vi "Main.vi"() -> ()   [LabVIEW 2017]
doc: "This Continuous Measurement sample project is based on the Queued Message Handler template.\n\nThe Event Handling Loop generates messages based on user interface actions.\n\nThe Message Handling Loop processes messages generated by the Event Handling Loop, or by other messages. There are also Acquisition and Logging message handling loop subVIs, and a chart updating loop."
uses:
  Settings/Settings.ctl
  Acquisition/Hardware Configuration.ctl
  Acquisition/Signal Type.ctl
  Logging/Logging Configuration.ctl
  controls/UI Data.ctl
  controls/UI State.ctl
  support/Message Queue/Enqueue Message (Single).vi
  controls/ExitGlobal.vi
  support/Message Queue/Enqueue Message (Array).vi
  <vilib>/Utility/error.llb/Error Cluster From Error Code.vi
  <vilib>/ErrorRing/Error Ring.xnode
  Acquisition/Acquisition.lvlib
  Logging/Logging.lvlib
  Settings/Settings.lvlib
  support/User Event - Stop/User Event - Stop.lvlib
  support/Message Queue/Message Queue.lvlib
  Settings/Settings Dialog.vi
panel:
  out "Zero run":bool
  in  "Zero run?":bool
  out "Max writing time to a file [min]":dbl
  out "Test time zero run [s]":dbl
  out "Test time [s]":dbl
  in  "Start":bool
  in  "Stop":bool
  in  "Settings":bool
  out "Status":string
  in  "Exit":bool
  out "Log File Offsite Path":path
  out "Project code":string
  out "Offsite storage?":bool
  out "Log File Path":path
  out "Data":waveform(dbl)[](graph)
  # "Continuous Measurement Data Logger"
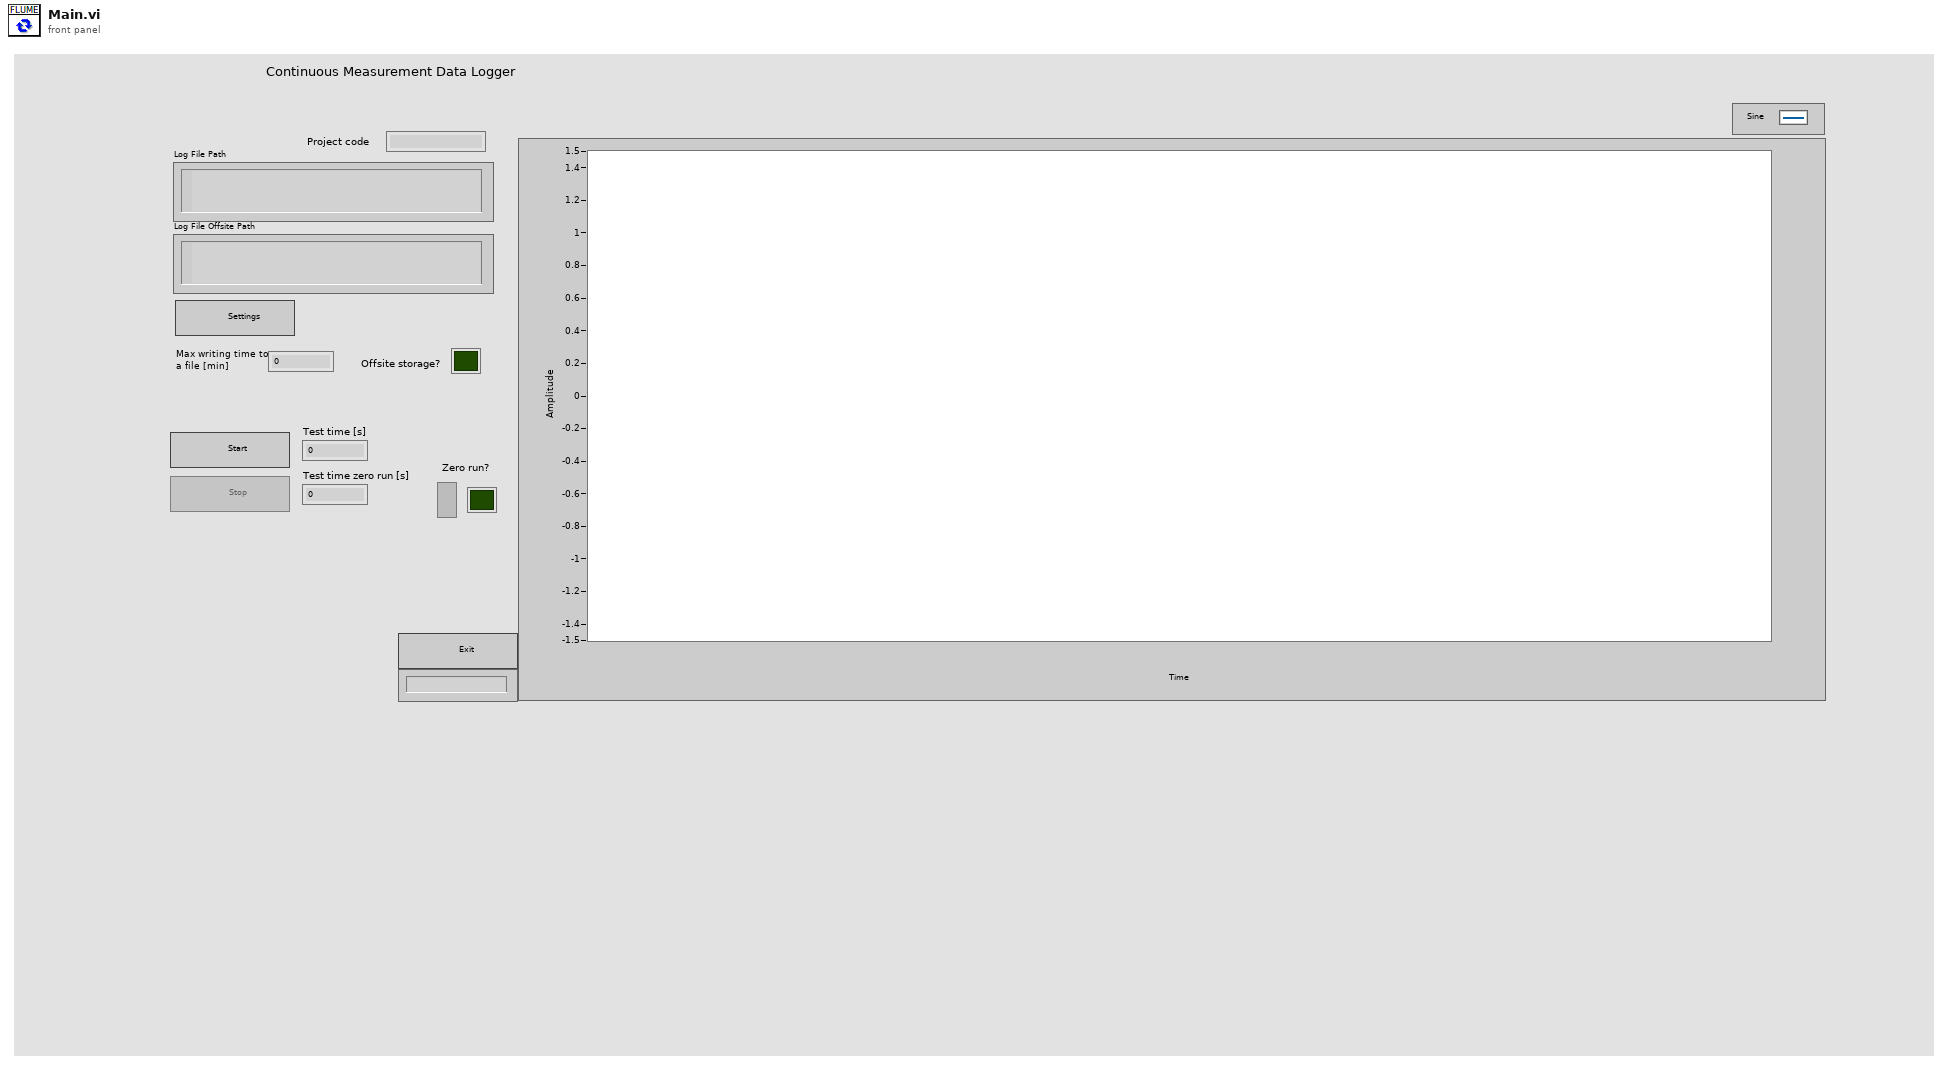
[diagram p1: front panel]
types:
  T1 = cluster{"Offsite storage?":bool, "Test time [s]":dbl, "Test time zero run [s] ":dbl, "Max writing time to a file [min]":dbl, "Zero run":bool}
  T2 = typedef "UI State.ctl" = enum16{"Idle", "Acquiring and Logging", "Waiting for Exit", "Waiting for Exit (Acq Stopped)", "Waiting for Exit (Log Stopped)", "Waiting for Stop", "Waiting for Stop (Acq Stopped)", "Waiting for Stop (Log Stopped)"}
  T3 = typedef "UI Data.ctl" = cluster{"Start Ref":refnum<vi>, "Stop Ref":refnum<vi>, "Settings Ref":refnum<vi>, "Exit Ref":refnum<vi>, "Status Ref":refnum<vi>, "Data Ref":refnum<vi>, "Zero run Ref":refnum<vi>}
  T4 = typedef "Settings.lvlib/Settings.ctl" = cluster{"Hardware Configuration":T5, "Logging Configuration":T7, "Timers":cluster{"Offsite storage?":bool, "Test time [s]":dbl, "Test time zero run [s] ":dbl, "Max writing time to a file [min]":dbl, "Zero run":bool}}
  T5 = typedef "Acquisition.lvlib/Hardware Configuration.ctl" = cluster{"HW Refnum <Replace Me>":string, "Signal Type <Replace Me>":T6}
  T6 = typedef "Acquisition.lvlib/Signal Type.ctl" = enum16{"Sine Wave", "Square with Noise"}
  T7 = typedef "Logging.lvlib/Logging Configuration.ctl" = cluster{"Log File Base Path":path, "TDMS File Reference":refnum<k34>, "Log File Offsite Path":path, "Project code":string, "Bin File Reference":refnum<file>}
  T8 = typedef "Message Queue.lvlib/All Message Queues.ctl" = cluster{"UI":refnum<queue>, "Acquisition":refnum<queue>, "Logging":refnum<queue>, "Bin Logging":refnum<queue>, "Time":refnum<queue>}
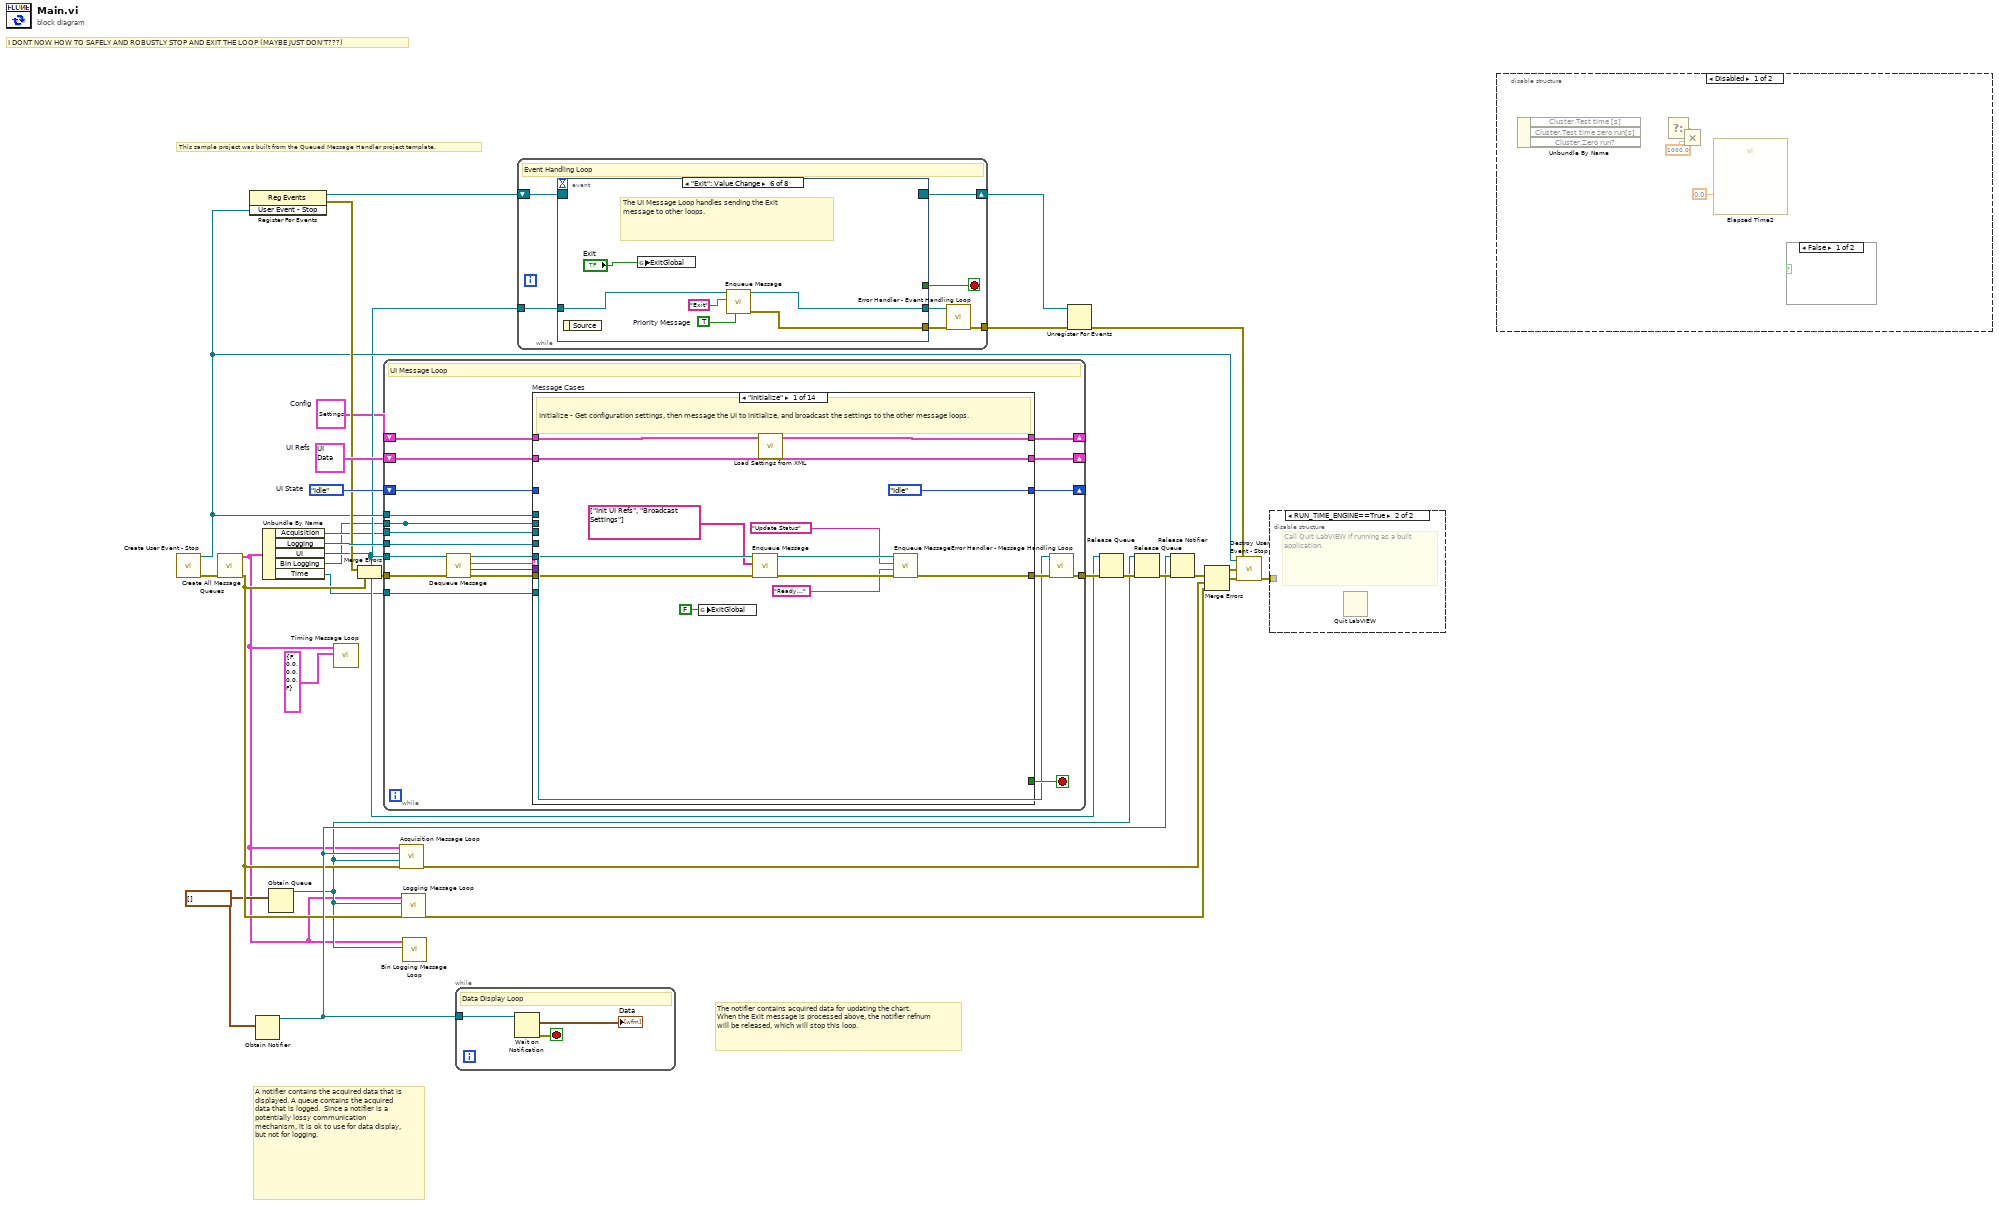
[diagram p0: block diagram]
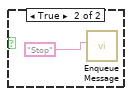
[diagram p2: hidden frame]
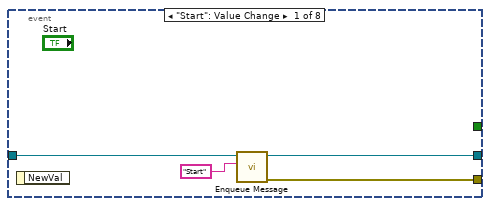
[diagram p5: hidden frame]
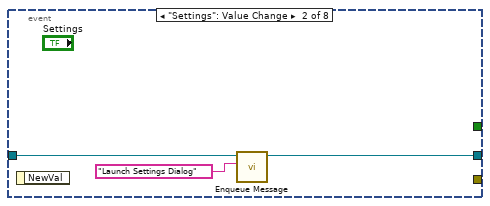
[diagram p6: hidden frame]
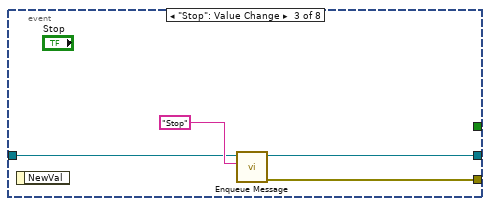
[diagram p7: hidden frame]
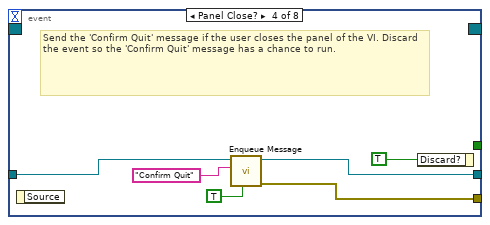
[diagram p8: hidden frame]
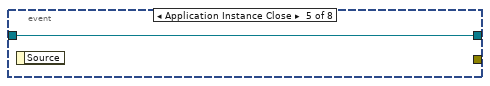
[diagram p9: hidden frame]
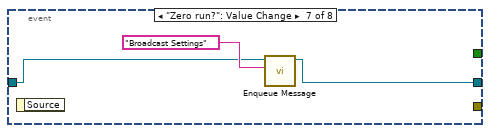
[diagram p10: hidden frame]
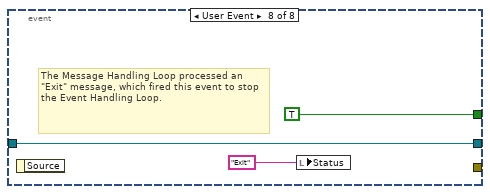
[diagram p11: hidden frame]
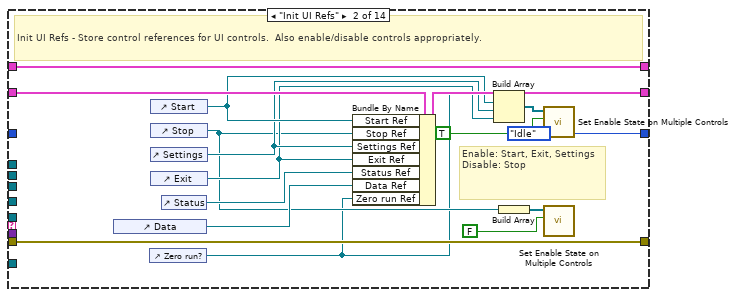
[diagram p12: hidden frame]
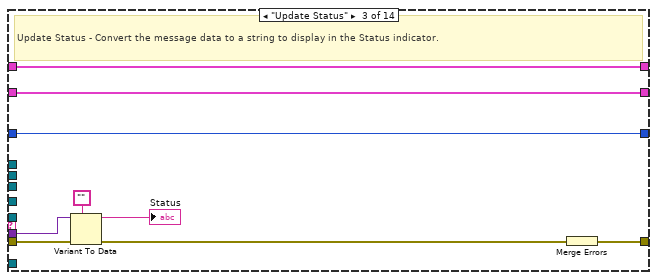
[diagram p13: hidden frame]
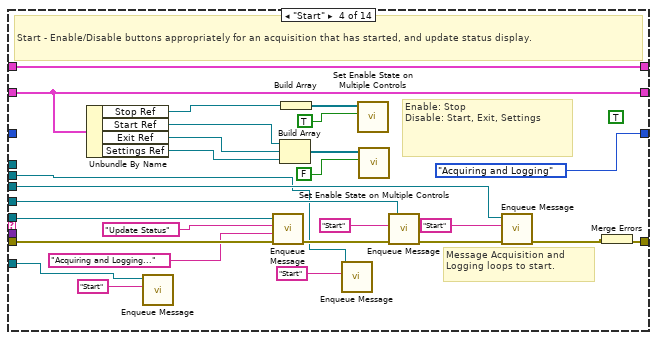
[diagram p14: hidden frame]
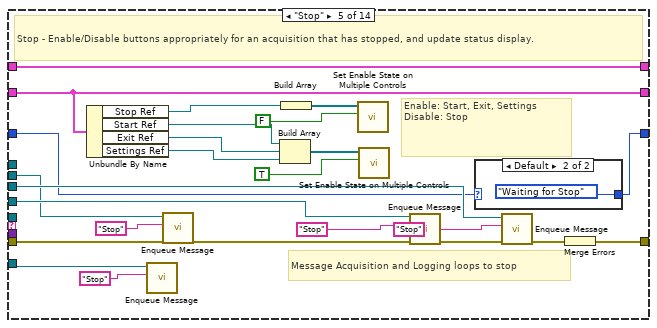
[diagram p15: hidden frame]
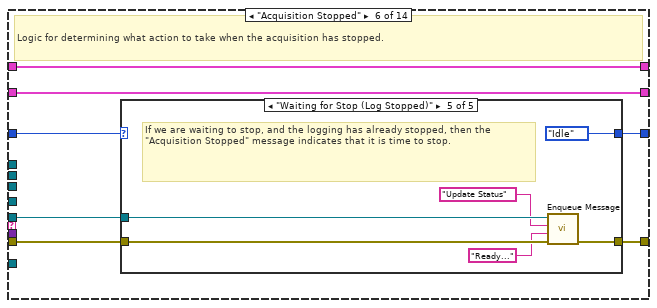
[diagram p17: hidden frame]
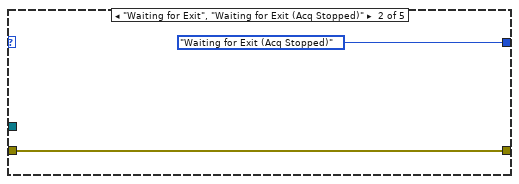
[diagram p19: hidden frame]
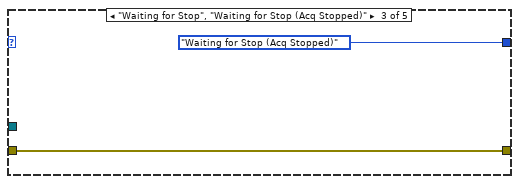
[diagram p20: hidden frame]
diagram:
  w23 = UI_State."Idle"  # UI State
  w7 = waveform(dbl)[] []
  w25 = T3 {"Start Ref"=refnum, "Stop Ref"=refnum, "Settings Ref"=refnum, "Exit Ref"=refnum, "Status Ref"=refnum, "Data Ref"=refnum, "Zero run Ref"=refnum}  # UI Refs
  w9 = T4 {"Hardware Configuration"={"HW Refnum <Replace Me>"="", "Signal Type <Replace Me>"=enum."Sine Wave"}, "Logging Configuration"={"Log File Base Path"=path "", "TDMS File Reference"=refnum, "Log File Offsite Path"=path "", "Project code"="", "Bin File Reference"=refnum}, "Timers"={"Offsite storage?"=FALSE, "Test time [s]"=10.0, "Test time zero run [s] "=180.0, "Max writing time to a file [min]"=30.0, "Zero run"=FALSE}}  # Config
  # "I DONT NOW HOW TO SAFELY AND ROBUSTLY STOP AND EXIT THE LOOP (MAYBE JUST DON'T???)"
  # "This sample project was built from the Queued Message Handler project template."
  # "A notifier contains the acquired data that is displayed. A queue contains the acquired data that is logged.  Since a notifier is a potentially lossy communication mechanism, it is ok to use for data display, but not for logging."
  # "The notifier contains acquired data for updating the chart. When the Exit message is processed above, the notifier refnum will be released, which will stop this loop."
  n1 = call "Create User Event - Stop.vi"() -> ("error out"=w27:errorcluster, "User Event - Stop"=w14:refnum<user-event>)  [unwired: 10 in]
  n2 = call "Create All Message Queues.vi"("error in (no error)"=w27) -> ("error out"=w8:errorcluster, "Message Queues out"=w2:T8)  [unwired: 9 in]
  n3 = register-events(w14) -> (reference out=w17:refnum<event-registration>, error out=w15:errorcluster)  [unwired: 2 in]
  n4 = Obtain Notifier(notification data type=w7) -> (notifier out=w10:refnum<notifier>)  [unwired: 3 in, 2 out]
  n5 = Unbundle By Name(w2) -> ("Acquisition"=w12:refnum<queue>, "Logging"=w24:refnum<queue>, "UI"=w13:refnum<queue>, "Bin Logging"=w5:refnum<queue>, "Time"=w1:refnum<queue>)
  n6 = Obtain Queue(element data type=w7) -> (queue out=w6:refnum<queue>)  [unwired: 4 in, 2 out]
  n7 = call "Timing Message Loop.vi"("Timers"=T1 {"Offsite storage?"=FALSE, "Test time [s]"=0.0, "Test time zero run [s] "=0.0, "Max writing time to a file [min]"=0.0, "Zero run"=FALSE}, "Message Queues"=w2) -> ()  [unwired: 9 in, 1 out]
  n8 = Merge Errors(w15, w8) -> (w16:errorcluster)
  n9 = while {
    tunnel: w13 -> [w36]
    tunnel: w14 -> [w49]
    shift-right: [w44] -> _
    shift-left: w9 -> [w32]
    shift-right: [w42] -> _
    shift-left: w25 -> [w43]
    tunnel: w12 -> [w41]
    tunnel: w24 -> [w35]
    shift-right: [w37] -> _
    shift-left: w23 -> [w38]
    tunnel: w16 -> [w48]
    tunnel: [w40] -> w30
    tunnel: w5 -> [w33]
    tunnel: [w33] -> _
    tunnel: w1 -> [w31]
    stop <- w50 stop-if-true
    # "UI Message Loop"
    n10 = call "Dequeue Message.vi"("error in (no error)"=w48, "Message Queue"=w36) -> ("error out"=w47:errorcluster, "Message Data"=w45:variant, "Message"=w46:string, "dup Message Queue"=w34:refnum<queue>)  [unwired: 6 in]
    n11 = case "Message Cases" shown="\"Initialize\"" w46 {
      selector: w46 -> [_ _ _ _ _ _ _ _ _ _ _ _ _ w295]
      tunnel: w34 -> [w56 _ _ w94 _ w145 w170 _ w223 _ w245 _ _ _]
      tunnel: w47 -> [w55 w79 w87 w115 w138 w146 w171 w213 w225 w233 w244 w279 w293 _]
      tunnel: [w60 w79 w88 w96 w139 w143 w168 w217 w219 w236 w243 w286 w292 w294] -> w39
      tunnel: [_ _ _ _ _ _ _ _ _ _ _ TRUE _ _] -> w50
      tunnel: w45 -> [_ _ w86 _ _ _ _ _ _ w237 _ w277 _ _]
      tunnel: w49 -> [_ _ _ _ _ _ _ _ _ _ _ w287 _ _]
      tunnel: [w63 w66 w80 w92 w120 w142 w167 w196 w218 w232 w241 w275 w291 w298] -> w44
      tunnel: w32 -> [w52 w66 w80 w92 w120 w142 w167 w201 w226 w232 w241 w275 w291 w298]
      tunnel: w43 -> [w57 w78 w82 w112 w137 w148 w173 w212 w221 w240 w247 w285 w290 w297]
      tunnel: [w57 w75 w82 w112 w137 w148 w173 w212 w221 w240 w247 w285 w290 w297] -> w42
      tunnel: w41 -> [_ _ _ w95 w124 _ _ w211 _ _ _ w284 _ _]
      tunnel: w35 -> [_ _ _ w101 w127 _ _ w210 _ _ _ w283 _ _]
      tunnel: w38 -> [_ _ w81 _ w121 w147 w172 w209 w220 w235 w246 _ w289 w296]
      tunnel: [UI_State."Idle" ("UI State") UI_State."Idle" ("UI State") w81 UI_State."Acquiring and Logging" ("UI State") w122 w144 w169 w209 w220 w235 w242 UI_State."Idle" ("UI State") w289 w296] -> w37
      tunnel: w33 -> [_ _ _ w91 w118 _ _ w204 _ _ _ w274 _ _]
      tunnel: w31 -> [_ _ _ w89 w117 _ _ w200 _ _ _ w270 _ _]
      frame "Initialize" {
        # "Initialize - Get configuration settings, then message the UI to initialize, and broadcast the settings to the other message loops."
        n12 = global write "ExitGlobal.vi" "ExitGlobal"(FALSE ("ExitGlobal")) -> ()
        n13 = call-poly "Enqueue Message.vi"("error in (no error)"=w55, "Message Array"=string[] ["Init UI Refs", "Broadcast Settings"], "Message Queue"=w56) -> ("error out"=w62:errorcluster, "dup Message Queue"=w61:refnum<queue>)  [unwired: 7 in]
        n14 = call "Load Settings from XML.vi"("Settings in"=w52) -> ("Settings out"=w63:T4)  [unwired: 9 in, 1 out]
        n15 = call-poly "Enqueue Message.vi"("error in (no error)"=w62, "Message Data"="Ready..." ("Ready..."), "Message"="Update Status", "Message Queue"=w61) -> ("error out"=w60:errorcluster)  [unwired: 6 in, 1 out]
      }
      frame "Init UI Refs" {
        # "Enable: Start, Exit, Settings\nDisable: Stop"
        # "Init UI Refs - Store control references for UI controls.  Also enable/disable controls appropriately."
        n16 = control-ref of="Data"() -> (w76:refnum<vi>)
        n17 = control-ref of="Zero run?"() -> (w64:refnum<vi>)
        n18 = control-ref of="Start"() -> (w70:refnum<vi>)
        n19 = control-ref of="Stop"() -> (w65:refnum<vi>)
        n20 = control-ref of="Settings"() -> (w69:refnum<vi>)
        n21 = control-ref of="Exit"() -> (w68:refnum<vi>)
        n22 = control-ref of="Status"() -> (w77:refnum<vi>)
        n23 = Bundle By Name(cluster=w78, "Start Ref"=w70, "Stop Ref"=w65, "Settings Ref"=w69, "Exit Ref"=w68, "Status Ref"=w77, "Data Ref"=w76, "Zero run Ref"=w64) -> (w75:T3)
        n24 = Build Array(w64, w70, w69, w68) -> (w73:refnum<vi>[])
        n25 = Build Array(w65) -> (w72:refnum<vi>[])
        n26 = call "Set Enable State on Multiple Controls.vi"("Enable?"=TRUE, "Controls"=w73) -> ()  [unwired: 10 in]
        n27 = call "Set Enable State on Multiple Controls.vi"("Enable?"=FALSE, "Controls"=w72) -> ()  [unwired: 10 in]
      }
      frame "Update Status" {
        # "Update Status - Convert the message data to a string to display in the Status indicator."
        n28 = Variant To Data(error in=w87, type="", Variant=w86) -> (data=→"Status":string, error out=w84:errorcluster)
        n29 = Merge Errors(w84) -> (w88:errorcluster)
      }
      frame "Start" {
        (unwired) TRUE ("Reset")
        # "Message Acquisition and Logging loops to start."
        # "Enable: Stop\nDisable: Start, Exit, Settings"
        # "Start - Enable/Disable buttons appropriately for an acquisition that has started, and update status display."
        n30 = Unbundle By Name(w112) -> ("Stop Ref"=w107:refnum<vi>, "Start Ref"=w106:refnum<vi>, "Exit Ref"=w105:refnum<vi>, "Settings Ref"=w104:refnum<vi>)
        n31 = call-poly "Enqueue Message.vi"("Message"="Start", "Message Queue"=w89) -> ()  [unwired: 8 in, 2 out]
        n32 = call-poly "Enqueue Message.vi"("error in (no error)"=w115, "Message Data"="Acquiring and Logging..." ("Acquiring and Logging..."), "Message"="Update Status", "Message Queue"=w94) -> ("error out"=w103:errorcluster)  [unwired: 6 in, 1 out]
        n33 = Build Array(w106, w105, w104) -> (w110:refnum<vi>[])
        n34 = Build Array(w107) -> (w109:refnum<vi>[])
        n35 = call-poly "Enqueue Message.vi"("Message"="Start", "Message Queue"=w91) -> ()  [unwired: 8 in, 2 out]
        n36 = call "Set Enable State on Multiple Controls.vi"("Enable?"=TRUE, "Controls"=w109) -> ()  [unwired: 10 in]
        n37 = call "Set Enable State on Multiple Controls.vi"("Enable?"=FALSE, "Controls"=w110) -> ()  [unwired: 10 in]
        n38 = call-poly "Enqueue Message.vi"("error in (no error)"=w103, "Message"="Start", "Message Queue"=w101) -> ("error out"=w98:errorcluster)  [unwired: 7 in, 1 out]
        n39 = call-poly "Enqueue Message.vi"("error in (no error)"=w98, "Message"="Start", "Message Queue"=w95) -> ("error out"=w97:errorcluster)  [unwired: 7 in, 1 out]
        n40 = Merge Errors(w97) -> (w96:errorcluster)
      }
      frame "Stop" {
        # "Message Acquisition and Logging loops to stop"
        # "Enable: Start, Exit, Settings\nDisable: Stop"
        # "Stop - Enable/Disable buttons appropriately for an acquisition that has stopped, and update status display."
        n41 = Unbundle By Name(w137) -> ("Stop Ref"=w132:refnum<vi>, "Start Ref"=w131:refnum<vi>, "Exit Ref"=w130:refnum<vi>, "Settings Ref"=w129:refnum<vi>)
        n42 = call-poly "Enqueue Message.vi"("Message"="Stop", "Message Queue"=w117) -> ()  [unwired: 8 in, 2 out]
        n43 = call-poly "Enqueue Message.vi"("Message"="Stop", "Message Queue"=w118) -> ()  [unwired: 8 in, 2 out]
        n44 = Build Array(w131, w130, w129) -> (w135:refnum<vi>[])
        n45 = Build Array(w132) -> (w134:refnum<vi>[])
        n46 = call "Set Enable State on Multiple Controls.vi"("Enable?"=FALSE, "Controls"=w134) -> ()  [unwired: 10 in]
        n47 = call "Set Enable State on Multiple Controls.vi"("Enable?"=TRUE, "Controls"=w135) -> ()  [unwired: 10 in]
        n48 = call-poly "Enqueue Message.vi"("error in (no error)"=w138, "Message"="Stop", "Message Queue"=w127) -> ("error out"=w126:errorcluster)  [unwired: 7 in, 1 out]
        n49 = case shown="Default" w121 {
          selector: w121 -> [w140 _]
          tunnel: [w140 UI_State."Waiting for Stop" ("UI State")] -> w122
          frame "Waiting for Exit" {
          }
          frame Default {
          }
        }
        n50 = call-poly "Enqueue Message.vi"("error in (no error)"=w126, "Message"="Stop", "Message Queue"=w124) -> ("error out"=w125:errorcluster)  [unwired: 7 in, 1 out]
        n51 = Merge Errors(w125) -> (w139:errorcluster)
      }
      frame "Acquisition Stopped" {
        # "Logic for determining what action to take when the acquisition has stopped."
        n52 = case shown="\"Waiting for Stop (Log Stopped)\"" w147 {
          selector: w147 -> [w150 _ _ _ _]
          tunnel: w146 -> [w149 w152 w154 w160 w166]
          tunnel: w145 -> [_ _ _ w158 w163]
          tunnel: [w150 UI_State."Waiting for Exit (Acq Stopped)" ("UI State") UI_State."Waiting for Stop (Acq Stopped)" ("UI State") UI_State."Idle" ("UI State") UI_State."Idle" ("UI State")] -> w144
          tunnel: [w149 w152 w154 w159 w164] -> w143
          frame Default {
          }
          frame "Waiting for Exit", "Waiting for Exit (Acq Stopped)" {
          }
          frame "Waiting for Stop", "Waiting for Stop (Acq Stopped)" {
          }
          frame "Waiting for Exit (Log Stopped)" {
            # "If we are waiting to exit, and the logging has already stopped, then the \"Acquisition Stopped\" message indicates that it is time to exit."
            n53 = call-poly "Enqueue Message.vi"("Priority Message? (F)"=TRUE, "error in (no error)"=w160, "Message"="Exit", "Message Queue"=w158) -> ("error out"=w159:errorcluster)  [unwired: 6 in, 1 out]
          }
          frame "Waiting for Stop (Log Stopped)" {
            # "If we are waiting to stop, and the logging has already stopped, then the \"Acquisition Stopped\" message indicates that it is time to stop."
            n54 = call-poly "Enqueue Message.vi"("error in (no error)"=w166, "Message Data"="Ready..." ("Ready..."), "Message"="Update Status", "Message Queue"=w163) -> ("error out"=w164:errorcluster)  [unwired: 6 in, 1 out]
          }
        }
      }
      frame "Logging Stopped" {
        # "Logic for determining what action to take when the logging has stopped."
        n55 = case shown="Default" w172 {
          selector: w172 -> [w175 _ _ _ _]
          tunnel: w171 -> [w174 w177 w179 w185 w188]
          tunnel: w170 -> [_ _ _ w183 w187]
          tunnel: [w175 UI_State."Waiting for Exit (Log Stopped)" ("UI State") UI_State."Waiting for Stop (Log Stopped)" ("UI State") UI_State."Idle" ("UI State") UI_State."Idle" ("UI State")] -> w169
          tunnel: [w174 w177 w179 w184 w186] -> w168
          frame Default {
          }
          frame "Waiting for Exit", "Waiting for Exit (Log Stopped)" {
          }
          frame "Waiting for Stop", "Waiting for Stop (Log Stopped)" {
          }
          frame "Waiting for Exit (Acq Stopped)" {
            # "If we are waiting to exit, and the acquisition has already stopped, then the \"Logging Stopped\" message indicates that it is time to exit."
            n56 = call-poly "Enqueue Message.vi"("Priority Message? (F)"=TRUE, "error in (no error)"=w185, "Message"="Exit", "Message Queue"=w183) -> ("error out"=w184:errorcluster)  [unwired: 6 in, 1 out]
          }
          frame "Waiting for Stop (Acq Stopped)" {
            # "If we are waiting to stop, and the acquisition has already stopped, then the \"Logging Stopped\" message indicates that it is time to stop."
            n57 = call-poly "Enqueue Message.vi"("error in (no error)"=w188, "Message Data"="Ready..." ("Ready..."), "Message"="Update Status", "Message Queue"=w187) -> ("error out"=w186:errorcluster)  [unwired: 6 in, 1 out]
          }
        }
      }
      frame "Broadcast settings" {
        w199 = "Update Settings" ("Message")
        # "Broadcast settings - Send the 'Update Settings' message to the Logging and Acquisition message loops."
        n58 = Unbundle By Name(w201) -> ("Hardware Configuration"=w215:T5, "Logging Configuration"=w203:T7, "Timers"=w198:T1)
        n59 = Unbundle By Name(w203) -> ("Log File Base Path"=→"Log File Path":path, "Log File Offsite Path"=→"Log File Offsite Path":path, "Project code"=→"Project code":string)
        n60 = Bundle By Name(cluster=w201, "Timers.Zero run"="Zero run?") -> (w196:T4)
        n61 = Unbundle By Name(w198) -> ("Max writing time to a file [min]"=→"Max writing time to a file [min]":dbl, "Offsite storage?"=→"Offsite storage?":bool, "Test time [s]"=→"Test time [s]":dbl, "Test time zero run [s]"=→"Test time zero run [s]":dbl)
        n62 = Unbundle By Name(w196) -> ("Timers"=w195:T1)
        n63 = call-poly "Enqueue Message.vi"("Message Data"=w215, "Message"=w199, "Message Queue"=w211) -> ("error out"=w216:errorcluster)  [unwired: 7 in, 1 out]
        n64 = call-poly "Enqueue Message.vi"("Message Data"=w195, "Message"=w199, "Message Queue"=w200) -> ("error out"=w194:errorcluster)  [unwired: 7 in, 1 out]
        n65 = call-poly "Enqueue Message.vi"("Message Data"=w203, "Message"=w199, "Message Queue"=w204) -> ()  [unwired: 7 in, 2 out]
        n66 = call-poly "Enqueue Message.vi"("error in (no error)"=w216, "Message Data"=w203, "Message"=w199, "Message Queue"=w210) -> ("error out"=w214:errorcluster)  [unwired: 6 in, 1 out]
        n67 = Merge Errors(w214, w213, w194) -> (w217:errorcluster)
        "Zero run" <- "Zero run?"
      }
      frame "Launch Settings Dialog" {
        # "Launch Settings Dialog - Launch the Settings Dialog when the user clicks the 'Settings' button."
        n68 = call-by-ref "?"("error in (no error)"=w225, "Settings in"=w226) -> ("error out"=w222:errorcluster, "Cancelled?"=w224:bool, "Settings out"=w218:T4)  [unwired: 8 in, 3 out]
        n69 = case shown="False" w224 {
          tunnel: w223 -> [w230 _]
          tunnel: w222 -> [w229 w231]
          tunnel: [w228 w231] -> w219
          frame False {
            n70 = call-poly "Enqueue Message.vi"("error in (no error)"=w229, "Message"="Broadcast Settings", "Message Queue"=w230) -> ("error out"=w228:errorcluster)  [unwired: 7 in, 1 out]
          }
          frame True {
          }
        }
      }
      frame "Error" {
        # "Error - Display an error dialog. This message is sent by the \"Error Handler\" VIs at the end of other loops in this application."
        n71 = Variant To Data(error in=w233, type=errorcluster {"status"=FALSE, "code"=0, "source"=""} ("error constant"), Variant=w237) -> (data=w234:errorcluster, error out=w238:errorcluster)
        n72 = call <vilib>:"Simple Error Handler.vi"("error in (no error)"=w234) -> ()  [unwired: 4 in, 5 out]
        n73 = Merge Errors(w238) -> (w236:errorcluster)
      }
      frame "Confirm Quit" {
        # "Confirm Quit - Message that can confirm whether or not the user wants to exit the application."
        n74 = case shown="\"Acquiring and Logging\"" w246 {
          tunnel: w245 -> [w253 w257]
          tunnel: w244 -> [w252 w256]
          tunnel: [w251 w255] -> w243
          tunnel: [UI_State."Idle" ("UI State") w254] -> w242
          frame Default {
            # "If 'Confirm Quit' comes in while the system is idle, there is no need for a confirmation message."
            n75 = call-poly "Enqueue Message.vi"("Priority Message? (F)"=TRUE, "error in (no error)"=w252, "Message"="Exit", "Message Queue"=w253) -> ("error out"=w251:errorcluster)  [unwired: 6 in, 1 out]
          }
          frame "Acquiring and Logging" {
            n76 = Two Button Dialog(message="Are you sure you want to quit while the acquisition is running?" ("Confirm Quit Message"), 1:"No" ("No"), 2:"Yes" ("Yes")) -> (T button?=w258:bool)
            n77 = case shown="True" w258 {
              tunnel: w257 -> [_ w267]
              tunnel: w256 -> [w263 w268]
              tunnel: [w263 w266] -> w255
              tunnel: [UI_State."Acquiring and Logging" ("UI State") UI_State."Waiting for Exit" ("UI State")] -> w254
              frame False {
                # "User did not want to quit."
              }
              frame True {
                n78 = call-poly "Enqueue Message.vi"("error in (no error)"=w268, "Message"="Stop", "Message Queue"=w267) -> ("error out"=w266:errorcluster)  [unwired: 7 in, 1 out]
              }
            }
          }
        }
      }
      frame "Exit" {
        w280 = TRUE ("Priority Message? (F)")
        w273 = "Exit" ("Message")
        # "Popup an error dialog if 'Exit' was called as a result of an error."
        # "Stop the VI"
        # "Exit - Send Exit messages to the Acquisition and Logging loops, and fire the user event to stop the Event Handling Loop."
        n79 = call-poly "Enqueue Message.vi"("Message"="Exit", "Message Queue"=w270) -> ()  [unwired: 8 in, 2 out]
        n80 = Variant To Data(type=errorcluster {"status"=FALSE, "code"=0, "source"=""} ("error constant"), Variant=w277) -> (data=w276:errorcluster)  [unwired: 1 in, 1 out]
        n81 = call <vilib>:"Simple Error Handler.vi"("error in (no error)"=w276) -> ()  [unwired: 4 in, 5 out]
        n82 = call-poly "Enqueue Message.vi"("Priority Message? (F)"=w280, "error in (no error)"=w279, "Message"=w273, "Message Queue"=w284) -> ("error out"=w281:errorcluster)  [unwired: 6 in, 1 out]
        n83 = call-poly "Enqueue Message.vi"("Priority Message? (F)"=w280, "error in (no error)"=w281, "Message"=w273, "Message Queue"=w283) -> ("error out"=w272:errorcluster)  [unwired: 6 in, 1 out]
        n84 = call-poly "Enqueue Message.vi"("error in (no error)"=w272, "Message"=w273, "Message Queue"=w274) -> ("error out"=w271:errorcluster)  [unwired: 7 in, 1 out]
        n85 = call "Fire User Event - Stop.vi"("error in (no error)"=w271, "User Event - Stop"=w287) -> ("error out"=w286:errorcluster)  [unwired: 9 in]
      }
      frame "---Copy This Frame---" {
        (unwired) FALSE ("Time has Elapsed")
        # "Duplicate this frame when creating new messages.  Change this comment in the duplicated frame to describe this message."
        n86 = Merge Errors(w293) -> (w292:errorcluster)
      }
      frame Default {
        # "'Default' case only runs if there is a message that isn't defined in any of the other cases.  Output a programming error."
        n87 = xnode "Error Ring"("parameter 0"=w295) -> ("error out"=w294:errorcluster)
      }
    }
    n88 = call "Error Handler - Message Handling Loop.vi"("error in (no error)"=w39, "Message Queue"=w34) -> ("dup error in"=w40:errorcluster)  [unwired: 8 in, 1 out]
  }
  n89 = call "Acquisition Message Loop.vi"("error in (no error)"=w8, "Data Queue"=w6, "Data Notifier"=w10, "Message Queues"=w2) -> ("error out"=w28:errorcluster)  [unwired: 7 in]
  n90 = call "Logging Message Loop.vi"("error in (no error)"=w8, "Data Queue"=w6, "Message Queues"=w2) -> ("error out"=w4:errorcluster)  [unwired: 8 in]
  n91 = call "Bin Logging Message Loop.vi"("Data Queue"=w6, "Message Queues"=w2) -> ()  [unwired: 9 in, 1 out]
  n92 = while "Data Display Loop" {
    tunnel: w10 -> [w308]
    stop <- w307 stop-if-true
    # "Data Display Loop"
    n93 = Wait on Notification(notifier=w308) -> (notification=→"Data":waveform(dbl)[], error out=w307:errorcluster)  [unwired: 3 in, 2 out]
  }
  n94 = while {
    tunnel: w13 -> [w314]
    tunnel: [w311] -> w29
    shift-right: [w313] -> w26
    shift-left: w17 -> [w315]
    stop <- w312 stop-if-true
    # "Event Handling Loop"
    n95 = event shown="[5] \"Exit\": Value Change" {
      selector: w315 -> [_ _ _ _ _ _ _ _]
      dyn-events: [_ _ _ _ _ _ _ _] -> w313
      timeout: _ -> [_ _ _ _ _ _ _ _]
      tunnel: [_ _ _ _ _ _ _ TRUE ("Discard?")] -> w312
      tunnel: w314 -> [w319 w321 w325 w330 w333 w336 w341 w343]
      tunnel: [w317 _ w324 w328 _ w339 _ _] -> w310
      tunnel: [w316 w320 w323 w329 w333 w335 w340 w343] -> w309
      event "Start": Value Change {
        n96 = event-data() -> ()  [unwired: 1 in, 1 out]
        n97 = call-poly "Enqueue Message.vi"("Message"="Start", "Message Queue"=w319) -> ("error out"=w317:errorcluster, "dup Message Queue"=w316:refnum<queue>)  [unwired: 8 in]
      }
      event "Settings": Value Change {
        n98 = event-data() -> ()  [unwired: 1 in, 1 out]
        n99 = call-poly "Enqueue Message.vi"("Message"="Launch Settings Dialog", "Message Queue"=w321) -> ("dup Message Queue"=w320:refnum<queue>)  [unwired: 8 in, 1 out]
      }
      event "Stop": Value Change {
        n100 = event-data() -> ()  [unwired: 1 in, 1 out]
        n101 = call-poly "Enqueue Message.vi"("Message"="Stop", "Message Queue"=w325) -> ("error out"=w324:errorcluster, "dup Message Queue"=w323:refnum<queue>)  [unwired: 8 in]
      }
      event Panel Close? {
        # "Send the 'Confirm Quit' message if the user closes the panel of the VI. Discard the event so the 'Confirm Quit' message has a chance to run."
        n102 = event-data() -> ()  [unwired: 1 in, 1 out]
        n103 = call-poly "Enqueue Message.vi"("Priority Message? (F)"=TRUE, "Message"="Confirm Quit", "Message Queue"=w330) -> ("error out"=w328:errorcluster, "dup Message Queue"=w329:refnum<queue>)  [unwired: 7 in]
        n104 = event-data("Discard?"=TRUE) -> ()  [unwired: 1 in, 1 out]
      }
      event Application Instance Close {
        n105 = event-data() -> ()  [unwired: 1 in, 1 out]
      }
      event "Exit": Value Change {
        w337 = TRUE  # Priority Message
        # "The UI Message Loop handles sending the Exit message to other loops."
        n106 = event-data() -> ()  [unwired: 1 in, 1 out]
        n107 = global write "ExitGlobal.vi" "ExitGlobal"("Exit") -> ()
        n108 = call-poly "Enqueue Message.vi"("Priority Message? (F)"=w337, "Message"="Exit", "Message Queue"=w336) -> ("error out"=w339:errorcluster, "dup Message Queue"=w335:refnum<queue>)  [unwired: 7 in]
      }
      event "Zero run?": Value Change {
        n109 = event-data() -> ()  [unwired: 1 in, 1 out]
        n110 = call-poly "Enqueue Message.vi"("Message"="Broadcast Settings", "Message Queue"=w341) -> ("dup Message Queue"=w340:refnum<queue>)  [unwired: 8 in, 1 out]
      }
      event User Event {
        # "The Message Handling Loop processed an \"Exit\" message, which fired this event to stop the Event Handling Loop."
        n111 = event-data() -> ()  [unwired: 1 in, 1 out]
        n112 = local write "Status"("Exit" ("Exit String")) -> ()
      }
    }
    n113 = call "Error Handler - Event Handling Loop.vi"("error in (no error)"=w310, "Message Queue"=w309) -> ("dup error in"=w311:errorcluster)  [unwired: 8 in, 1 out]
  }
  n114 = Unregister For Events(event registration refnum=w26, error in=w29) -> (error out=w11:errorcluster)
  n115 = Release Queue(queue=w13, error in (no error)=w30) -> (error out=w20:errorcluster)  [unwired: 1 in, 2 out]
  n116 = Release Queue(queue=w6, error in (no error)=w20) -> (error out=w19:errorcluster)  [unwired: 1 in, 2 out]
  n117 = Release Notifier(notifier=w10, error in (no error)=w19) -> (error out=w18:errorcluster)  [unwired: 1 in, 2 out]
  n118 = Merge Errors(w11, w18, w28, w4) -> (w22:errorcluster)
  n119 = call "Destroy User Event - Stop.vi"("error in (no error)"=w22, "User Event - Stop"=w14) -> ("error out"=w21:errorcluster)  [unwired: 9 in]
  n120 = disable-structure shown="RUN_TIME_ENGINE==True" {
    disable-tunnel: w21 -> [_ _]
    frame condition #0 (active) {
    }
    frame condition #1 {
      # "Call Quit LabVIEW if running as a built application."
      n121 = Quit LabVIEW() -> ()  [unwired: 1 in]
    }
  }
  n122 = disable-structure shown="Disabled" {
    frame Disabled {
      n123 = Unbundle By Name() -> ()  [unwired: 1 in, 3 out]
      n124 = Select() -> (s? t:f=w348:dbl)  [unwired: 3 in]
      n125 = Multiply(x=w348, y=1000.0) -> ()  [unwired: 1 out]
      n126 = call "Elapsed Time2"("Set Start Time (s)"=0.0) -> ()  [unwired: 11 in, 8 out]
      n127 = case shown="False" {
        selector: _ -> [_ _]
        frame False {
        }
        frame True {
          n128 = call-poly "Enqueue Message.vi"("Message"="Stop") -> ()  [unwired: 9 in, 2 out]
        }
      }
    }
    frame Enabled {
    }
  }
